vi "New Data.vi"(8 "error in (no error)":errorcluster, 10 "New Data":T1, 11 "Data Logger Module in":refnum<class "Data Logger Module.lvclass">) -> (0 "error out":errorcluster, 3 "Data Logger Module out":refnum<class "Data Logger Module.lvclass">)   [LabVIEW 2020, in "VolatusData.lvlib" / "Data Logger Module.lvclass"]
uses:
  Data Logger Module.lvclass
  New Data.ctl
  Data Logger Module.lvclass/Data Logger Module.ctl
  VolatusData.lvlib
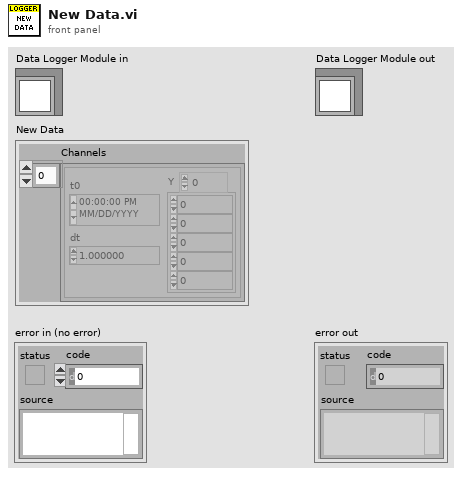
[diagram p1: front panel]
types:
  T1 = typedef "VolatusData.lvlib/New Data.ctl" = cluster{"Channels":waveform(dbl)[]}
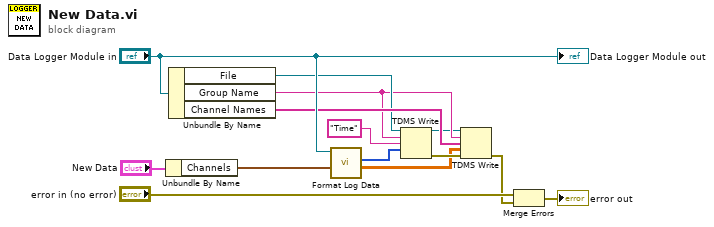
[diagram p0: block diagram]
diagram:
  n1 = Unbundle By Name("New Data") -> ("Channels"=w8:waveform(dbl)[])
  n2 = Unbundle By Name("Data Logger Module in") -> ("File"=w5:refnum<k34>, "Group Name"=w4:string, "Channel Names"=w6:string[])
  n3 = call "Format Log Data.vi"("Channels"=w8, "Data Logger Module in"="Data Logger Module in") -> ("Data"=w9:dbl[][], "Time"=w3:i64[])  [unwired: 6 in, 2 out]
  n4 = TDMS Write(0:w5, 5:w4, 7:"Time", 9:w3) -> (4:w1:refnum<k34>, 15:w14:errorcluster)  [unwired: 2 in, 2 out]
  n5 = TDMS Write(0:w1, 5:w4, 7:w6, 9:w9, 11:w14) -> (15:w10:errorcluster)  [unwired: 1 in, 3 out]
  n6 = Merge Errors("error in (no error)", w10) -> (→"error out":errorcluster)
  "Data Logger Module out" <- "Data Logger Module in"
